vi "PriorityColoring.vi"(7 "Array":u32[](array[colorbox]), 8 "Error In":errorcluster, 10 "Tbl Refnum":refnum<vi>, 11 "SR List In":T1[](array[typedef])) -> (0 "Error Out":errorcluster)   [LabVIEW 2017, in "Client.lvlib" / "UI_API.lvlib"]
uses:
  UI_API.lvlib
  ParserSorter/SR Data.ctl
  ParserSorter/AE Group.ctl
  ParserSorter/SR Status.ctl
  ParserSorter/SR Level.ctl
  ParserSorter/SR Type.ctl
  <vilib>/Utility/miscctls.llb/LVRowAndColumnTypeDef.ctl
  ParserSorter/ParserSorter.lvlib
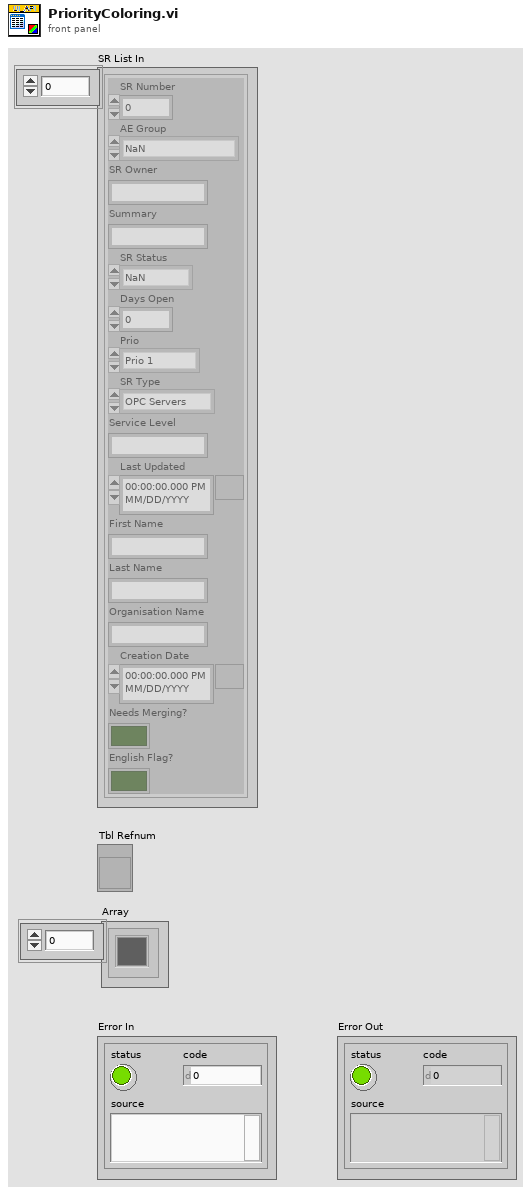
[diagram p1: front panel]
types:
  T1 = typedef "Client.lvlib/ParserSorter.lvlib/SR Data.ctl" = cluster{"SR Number":i64, "AE Group":T2, "SR Owner":string, "Summary":string, "SR Status":T3, "Days Open":dbl, "Prio":T4, "SR Type":T5, "Service Level":string, "Last Updated":timestamp, "First Name":string, "Last Name":string, "Organisation Name":string, "Creation Date":timestamp, "Needs Merging?":bool, "English Flag?":bool}
  T2 = typedef "Client.lvlib/ParserSorter.lvlib/AE Group.ctl" = enum32{"NaN", "AE-Germany", "AE-Poland", "AE-Switzerland", "AE-Czech Republic", "AE-Hungary", "AE-Romania", "AE-Slovakia", "AE-Slovenia"}
  T3 = typedef "Client.lvlib/ParserSorter.lvlib/SR Status.ctl" = enum32{"NaN", "Caller Abandoned", "Created in Error", "Declined to Purchase Support", "Expired", "Forum Resolved AE", "Forum Resolved Customer", "IN WORK", "IN WORK Collab with AES", "IN WORK Collab with PSE", "IN WORK Collab with SE", "IN WORK Escalation", "IN WORK Customer Added Note", "Open", "Potentially Resolved", "POC Resolved", "Resolved", "RMA Waiting on Customer", "RMA Open", "RMA In Progress", "RMA Closed - DOA", "RMA Closed", "RMA Approved for Return", "Project Complete", "Presumed Resolved", "IN WORK Wait on Customer"}
  T4 = typedef "Client.lvlib/ParserSorter.lvlib/SR Level.ctl" = enum16{"Prio 1", "Prio 2", "Prio 3", "Prio 4"}
  T5 = typedef "Client.lvlib/ParserSorter.lvlib/SR Type.ctl" = enum32{"NaN", "ATE Core Configurations (BYOATE)", "Activation", "BioBench", "CAN", "CM C Series", "Calibration", "Consulting Services", "CounterTimer", "DAQExpress", "DASYLab", "DIAdem", "DMM", "DSA HW", "Digital_IO", "FIRST (NIC Only)", "FieldBus", "FieldPoint", "Functional Savety", "GATI", "GPIB", "HMI and Industrial PCs", "HiQ", "HighSpeedDigital_IO", "IMAQ", "IOTech Vibration", "Industrial Communications", "InsightCM", "LV", "LV CD&Sim", "LV Comms", "LV Controls Add-Ons", "LV Embedded", "LV MathScript RT", "LV NXG", "LV NXT", "LVDSC", "LVFPGA", "LVPDA and LV Touch Panel", "LVRT", "LabWindows_CVI", "Lookout", "MATRIXx", "MStudioDotNet", "MStudioVisualBasic", "MStudioVisualC", "Measure (Legacy)", "Motion", "MultifunctionDAQ", "Multimedia Test HW/SW", "Multisim (EWB)", "NI Update Service", "OPC Servers", "Optical (OSI)", "PXI Controllers, Chassis, MXI", "PXI Timing and Sync", "Power Supplies and SMUs", "Powertrain Controls", "RAID", "RF", "RF Software", "RIO", "SC Express", "SCC", "SCXI", "SPEEDY-33 (Hyperception)", "STS", "ScopeDigitizers", "Serial", "Signal Sources", "SignalCondOther", "SignalExpress", "Software Defined Intruments", "Sound and Vibration SW", "Switch Executive", "Switches", "TestStand", "USRP", "Ultiboard (EWB)", "VBench", "VI Logger", "VXI_MXI", "VeriStand", "VisionSW", "VolumeLicenseMgr", "WSN", "Web UI Builder", "myRIO"}
  T6 = typedef "LVRowAndColumnTypeDef.ctl" = cluster{"Row":i32, "Column":i32}
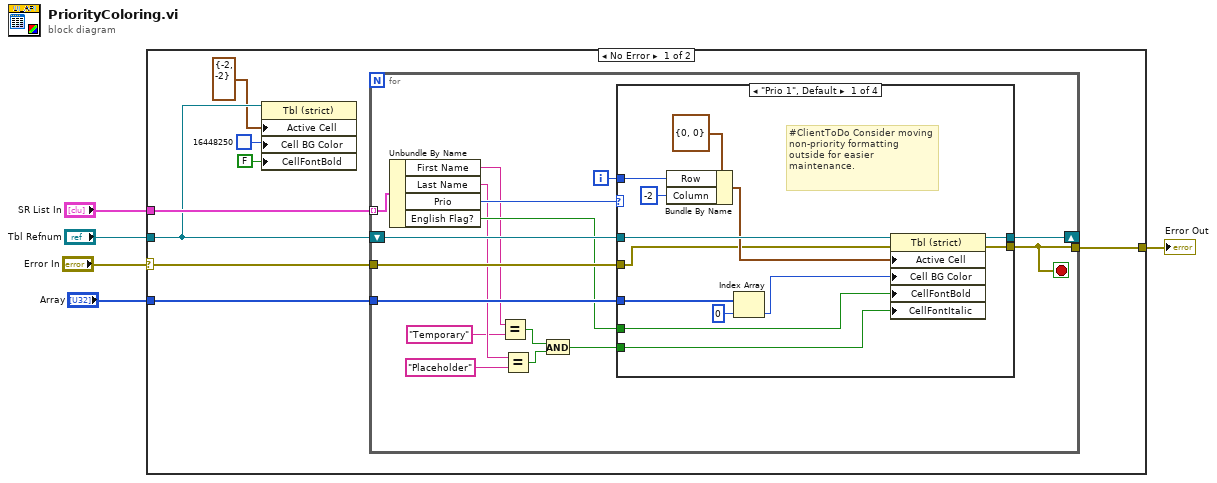
[diagram p0: block diagram]
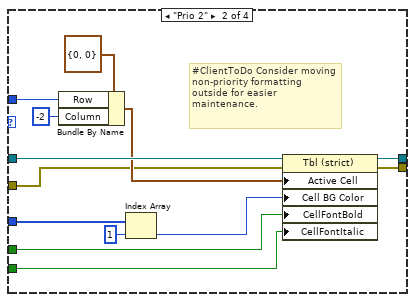
[diagram p2: hidden frame]
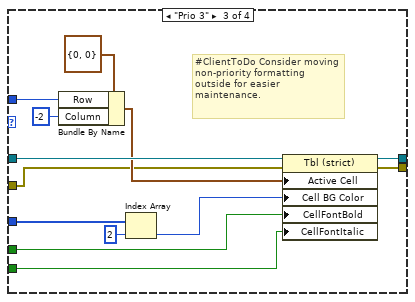
[diagram p3: hidden frame]
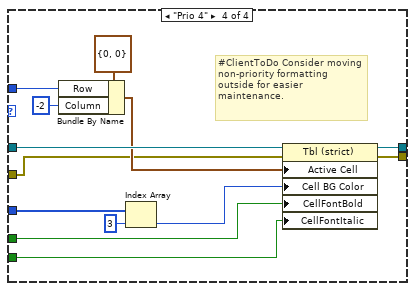
[diagram p4: hidden frame]
diagram:
  n1 = case shown="No Error" "Error In" {
    selector: "Error In" -> [w11 w82]
    tunnel: "SR List In" -> [w13 _]
    tunnel: "Tbl Refnum" -> [w9 _]
    tunnel: "Array" -> [w12 _]
    tunnel: [w10 w82] -> w1
    frame No Error {
      n2 = property class="Tbl (strict)"(reference=w9, "Active Cell"=T6 {"Row"=-2, "Column"=-2} ("Active Cell:Active Cell"), "Cell BG Color"=u32 16448250, "CellFontBold"=FALSE) -> ()  [unwired: 1 in, 2 out]
      n3 = for {
        tunnel: w13 -> [w29] mode=indexing
        tunnel: w12 -> [w27]
        shift-right: [w25] -> _
        shift-left: w9 -> [w28]
        tunnel: w11 -> [w24]
        tunnel: [w23] -> w10
        i -> [w26]
        stop <- w23 stop-if-true
        n4 = Unbundle By Name(w29) -> ("First Name"=w17:string, "Last Name"=w16:string, "Prio"=w22:T4, "English Flag?"=w21:bool)
        n5 = Equal?(x=w17, y="Temporary") -> (x = y?=w20:bool)
        n6 = Equal?(x=w16, y="Placeholder") -> (x = y?=w19:bool)
        n7 = And(x=w20, y=w19) -> (x .and. y?=w18:bool)
        n8 = case shown="\"Prio 1\", Default" w22 {
          tunnel: w28 -> [w42 w55 w68 w81]
          tunnel: w27 -> [w37 w50 w63 w76]
          tunnel: w26 -> [w40 w53 w66 w79]
          tunnel: [w34 w47 w60 w73] -> w25
          tunnel: w24 -> [w33 w46 w59 w72]
          tunnel: [w32 w45 w58 w71] -> w23
          tunnel: w21 -> [w31 w44 w57 w70]
          tunnel: w18 -> [w30 w43 w56 w69]
          frame "Prio 1", Default {
            # "#ClientToDo Consider moving non-priority formatting outside for easier maintenance."
            n9 = Bundle By Name(cluster=T6 {"Row"=0, "Column"=0} ("Active Cell:Active Cell"), "Row"=w40, "Column"=-2) -> (w38:T6)
            n10 = Index Array(array=w37, index=0) -> (element=w36:u32)
            n11 = property class="Tbl (strict)"(reference=w42, error in=w33, "Active Cell"=w38, "Cell BG Color"=w36, "CellFontBold"=w31, "CellFontItalic"=w30) -> (reference out=w34:refnum<vi>, error out=w32:errorcluster)
          }
          frame "Prio 2" {
            # "#ClientToDo Consider moving non-priority formatting outside for easier maintenance."
            n12 = Bundle By Name(cluster=T6 {"Row"=0, "Column"=0} ("Active Cell:Active Cell"), "Row"=w53, "Column"=-2) -> (w51:T6)
            n13 = Index Array(array=w50, index=1) -> (element=w49:u32)
            n14 = property class="Tbl (strict)"(reference=w55, error in=w46, "Active Cell"=w51, "Cell BG Color"=w49, "CellFontBold"=w44, "CellFontItalic"=w43) -> (reference out=w47:refnum<vi>, error out=w45:errorcluster)
          }
          frame "Prio 3" {
            # "#ClientToDo Consider moving non-priority formatting outside for easier maintenance."
            n15 = Bundle By Name(cluster=T6 {"Row"=0, "Column"=0} ("Active Cell:Active Cell"), "Row"=w66, "Column"=-2) -> (w64:T6)
            n16 = Index Array(array=w63, index=2) -> (element=w62:u32)
            n17 = property class="Tbl (strict)"(reference=w68, error in=w59, "Active Cell"=w64, "Cell BG Color"=w62, "CellFontBold"=w57, "CellFontItalic"=w56) -> (reference out=w60:refnum<vi>, error out=w58:errorcluster)
          }
          frame "Prio 4" {
            # "#ClientToDo Consider moving non-priority formatting outside for easier maintenance."
            n18 = Bundle By Name(cluster=T6 {"Row"=0, "Column"=0} ("Active Cell:Active Cell"), "Row"=w79, "Column"=-2) -> (w77:T6)
            n19 = Index Array(array=w76, index=3) -> (element=w75:u32)
            n20 = property class="Tbl (strict)"(reference=w81, error in=w72, "Active Cell"=w77, "Cell BG Color"=w75, "CellFontBold"=w70, "CellFontItalic"=w69) -> (reference out=w73:refnum<vi>, error out=w71:errorcluster)
          }
        }
      }
    }
    frame Error {
    }
  }
  "Error Out" <- w1
